vi "update.properties.request.vi"(8 "error in":errorcluster, 10 "properties":map{string, string}(c390), 11 "event":refnum<class "event.lvclass">) -> (0 "error out":errorcluster, 3 "request":string)   [LabVIEW 2020, in "event.lvclass"]
uses:
  event.lvclass
  event.lvclass/event.ctl
  13542d29-fea5-4531-aa33-706b80d0c749.vi
  <vilib>/JDP Science/JSONtext/Variant to JSON Text.vi
  <vilib>/JDP Science/JSONtext/support/Format JSON Object.vi
  <vilib>/JDP Science/JSONtext/LVClass Serializer/JSONtext LVClass Serializer.lvclass
  <vilib>/JDP Science/JSONtext/JSONtext.lvlib
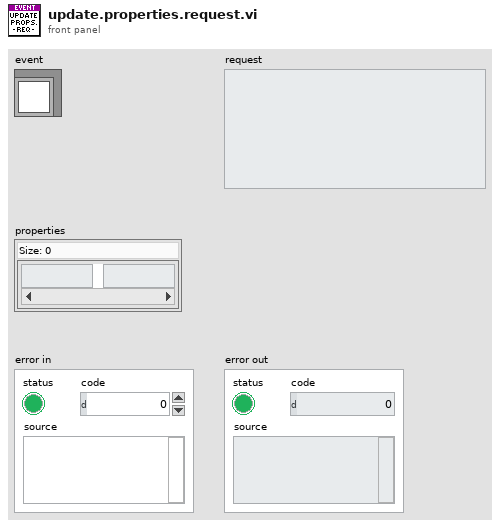
[diagram p1: front panel]
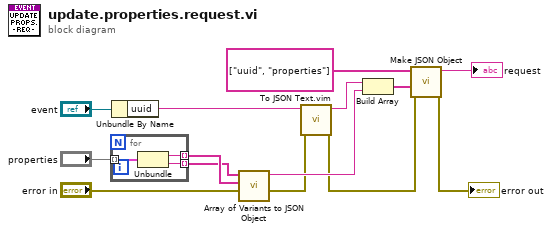
[diagram p0: block diagram]
diagram:
  n1 = for {
    tunnel: "properties" -> [w17] mode=indexing
    tunnel: [w16] -> w12 mode=indexing
    tunnel: [w15] -> w11 mode=indexing
    n2 = Unbundle(w17) -> ("name"=w16:string, "value"=w15:string)
  }
  n3 = Unbundle By Name("event") -> ("uuid"=w9:string)
  n4 = call <vilib>:"Array of Variants to JSON Object.vi"("error in (no error)"="error in", "Names"=w12, "Array"=w11) -> ("error out"=w3:errorcluster, "<JSON>"=w10:string)  [unwired: 7 in]
  n5 = call "To JSON Text.vim"("error in (no error)"=w3, "Anything"=w9) -> ("error out"=w4:errorcluster, "<JSON>"=w8:string)  [unwired: 8 in]
  n6 = Build Array(w8, w10) -> (w6:string[])
  n7 = call <vilib>:"Make JSON Object.vi"("error in (no error)"=w4, "JSON Items"=w6, "Item Names"=string[] ["uuid", "properties"]) -> ("error out"=→"error out":errorcluster, "<JSON>"=→"request":string)  [unwired: 7 in]
